vi "IPS Read PS Field.vi"(3 "Error In":errorcluster={"status"=FALSE, "code"=1073676294, "source"="VISA Read in Prologix USB GPIB Command.vi"}, 5 "VISA resource name (COM Port of Prologix Device)":refnum<visa-resource-name>="GPIB1::25::INSTR") -> (0 "Error Out":errorcluster={"status"=TRUE, "code"=85, "source"="Scan From String (arg 1) in IPS Read Field.vi->IV_B_2Gates_4461-4462.vi"}, 1 "Field (T)":dbl, 2 "VISA resource name (COM Port of Prologix Device) 2":refnum<visa-resource-name>)   [LabVIEW 2013]
panel:
  out "Error Out 2":errorcluster={"status"=TRUE, "code"=-1073807346, "source"="VISA Open in NI USB GPIB Command.vi->IPS Read Field.vi->IV_B_2Gates_4461-4462.vi"}
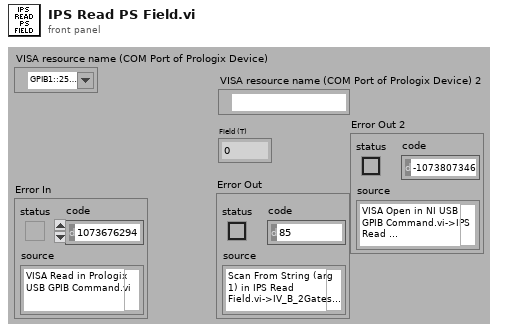
[diagram p1: front panel]
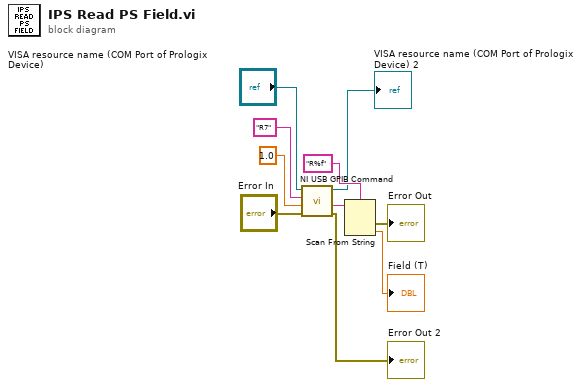
[diagram p0: block diagram]
diagram:
  n1 = call "NI USB GPIB Command.vi"("Error In"="Error In", "Wait for instrument to respond (s)"=1.0, "String to Send"="R7", "VISA resource name"="VISA resource name (COM Port of Prologix Device)") -> ("Error Out"=→"Error Out 2":errorcluster, "Return String from Device (Not all commands return a String)"=w6:string, "VISA resource name"=→"VISA resource name (COM Port of Prologix Device) 2":refnum<visa-resource-name>)  [unwired: 1 out]
  n2 = Scan From String(format string="R%f", input string=w6) -> (error out=→"Error Out":errorcluster, output 1=→"Field (T)":dbl)  [unwired: 2 in, 3 out]
